vi "team_name.vi"(8 "error in (no error)":errorcluster, 11 "Igor_1 in":refnum<class "Igor_1.lvclass">) -> (0 "error out":errorcluster, 2 "teamName":string, 3 "Igor_1 out":refnum<class "Igor_1.lvclass">)   [LabVIEW 2015, in "Igor_1.lvclass"]
uses:
  Igor_1.lvclass
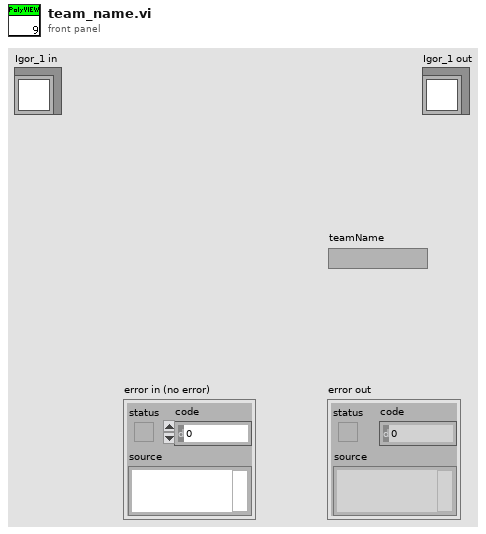
[diagram p1: front panel]
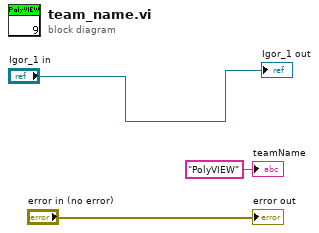
[diagram p0: block diagram]
diagram:
  "error out" <- "error in (no error)"
  "teamName" <- "PolyVIEW" ("teamName")
  "Igor_1 out" <- "Igor_1 in"
